vi "wrap error metadata.vi"(7 "additional info":string, 8 "error in (no error)":errorcluster, 9 "event name":string, 10 "task name":string, 11 "state name":string) -> (3 "error metadata":T1)   [LabVIEW 2024]
doc: "Description:\nThis VI generates an extended error metadata cluster (Error_Metadata) that combines the original error with contextual information such as task name, state name, event name, calling VI, timestamp, and additional custom info.\n\nUsage:\nCall this VI from any state or task within a QMH (Queued Message Handler) architecture when an error occurs. Provide the current task, state, and event names, along with any optional notes or extra context. The VI validates and formats the inputs, enriches the 'source' field of the original error, and returns a complete metadata cluster for logging or centralized error handling.\n\nInputs:\n- error in: The original LabVIEW error cluster.\n- task name, state name, event name, additional info: Contextual strings (validated internally).\n\nOutputs:\n- error metadata: Cluster containing error plus contextual metadata.\n- error out: The same error, with a modified source field for improved traceability.\n\nNotes:\n- Framework-agnostic: can be used with QMH, DQMH, Actor Framework, or custom architectures.\n- Especially useful for error routing to a central Error Handler loop.\n- Designed for scalability and readability in large applications."
uses:
  Error Wrapper.lvlib
  controls/error field names.ctl
  controls/error metadata.ctl
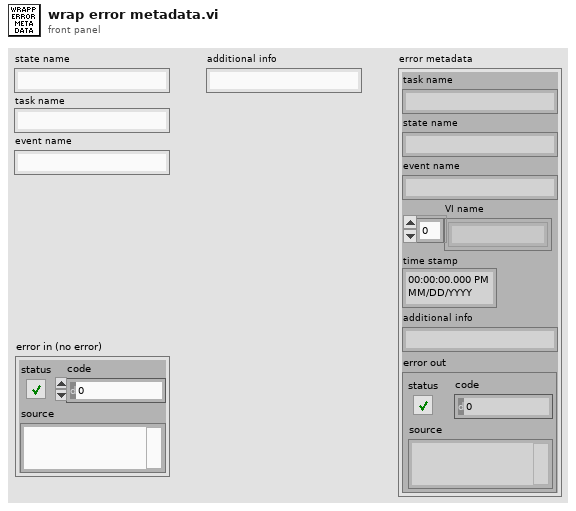
[diagram p1: front panel]
types:
  T1 = typedef "Error Wrapper.lvlib/error metadata.ctl" = cluster{"task name":string, "state name":string, "event name":string, "VI name":string[], "time stamp":timestamp, "additional info":string, "error out":errorcluster}
  T2 = typedef "Error Wrapper.lvlib/error field names.ctl" = enum32{"TASK NAME", "STATE NAME", "EVENT NAME", "ADDITIONAL INFO"}
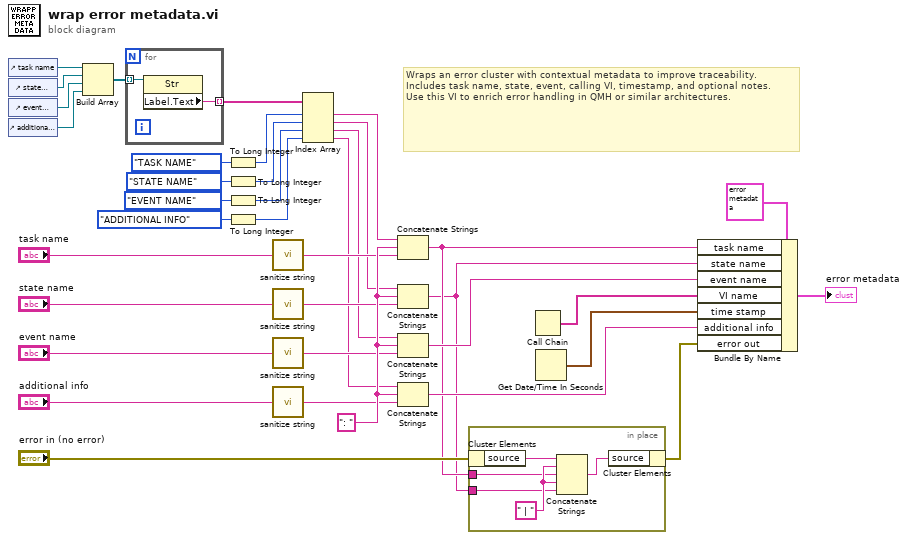
[diagram p0: block diagram]
diagram:
  w37 = ": "
  # "Wraps an error cluster with contextual metadata to improve traceability.\nIncludes task name, state, event, calling VI, timestamp, and optional notes.\nUse this VI to enrich error handling in QMH or similar architectures."
  n1 = control-ref of="task name"() -> (w22:refnum<vi>)
  n2 = control-ref of="state name"() -> (w21:refnum<vi>)
  n3 = control-ref of="event name"() -> (w20:refnum<vi>)
  n4 = control-ref of="additional info"() -> (w19:refnum<vi>)
  n5 = Build Array(w22, w21, w20, w19) -> (w18:refnum<vi>[])
  n6 = for {
    tunnel: w18 -> [w39] mode=indexing
    tunnel: [w38] -> w17 mode=indexing
    n7 = property on="Property Node" class="Str"(reference=w39) -> ("Label.Text"=w38:string)  [unwired: 1 in, 2 out]
  }
  n8 = To Long Integer(number=error_field_names."TASK NAME") -> (32bit integer=w11:i32)
  n9 = To Long Integer(number=error_field_names."STATE NAME") -> (32bit integer=w10:i32)
  n10 = To Long Integer(number=error_field_names."EVENT NAME") -> (32bit integer=w9:i32)
  n11 = To Long Integer(number=error_field_names."ADDITIONAL INFO") -> (32bit integer=w8:i32)
  n12 = call "sanitize string.vi"("string in"="task name") -> ("validated string"=w30:string)  [unwired: 4 in]
  n13 = call "sanitize string.vi"("string in"="state name") -> ("validated string"=w27:string)  [unwired: 4 in]
  n14 = call "sanitize string.vi"("string in"="event name") -> ("validated string"=w26:string)  [unwired: 4 in]
  n15 = call "sanitize string.vi"("string in"="additional info") -> ("validated string"=w24:string)  [unwired: 4 in]
  n16 = Index Array(array=w17, index #1=w11, index #2=w10, index #3=w9, index #4=w8) -> (element #1=w13:string, element #2=w14:string, element #3=w15:string, element #4=w16:string)
  n17 = Concatenate Strings(w13, w37, w30) -> (w2:string)
  n18 = Concatenate Strings(w14, w37, w27) -> (w1:string)
  n19 = Concatenate Strings(w15, w37, w26) -> (w32:string)
  n20 = Concatenate Strings(w16, w37, w24) -> (w31:string)
  n21 = in-place "In Place Element Structure" {
    in-place-border: w2 -> [w42]
    in-place-border: w1 -> [w41]
    w43 = " | "
    n22 = in-place-cluster #1("error in (no error)") -> ("source"=w44:string)
    n23 = Concatenate Strings(w44, w43, w42, w43, w41) -> (w40:string)
    n24 = in-place-cluster #1("source"=w40) -> (w3:errorcluster)
  }
  n25 = Call Chain() -> (call chain=w35:string[])
  n26 = Get Date/Time In Seconds() -> (seconds since 1Jan1904=w36:timestamp)
  n27 = Bundle By Name(cluster=T1 {"task name"="", "state name"="", "event name"="", "VI name"=[], "time stamp"=timestamp(0 s since 1904-01-01), "additional info"="", "error out"={"status"=FALSE, "code"=0, "source"=""}} ("error metadata"), "task name"=w2, "state name"=w1, "event name"=w32, "VI name"=w35, "time stamp"=w36, "additional info"=w31, "error out"=w3) -> (→"error metadata":T1)
